vi "ConfigFilePath.vi"(11 "Model Name":string) -> (3 "appended path":path)   [LabVIEW 2025, in "DAQ_Module.lvlib" / "DAQ_Module.lvclass"]
uses:
  DAQ_Module.lvclass
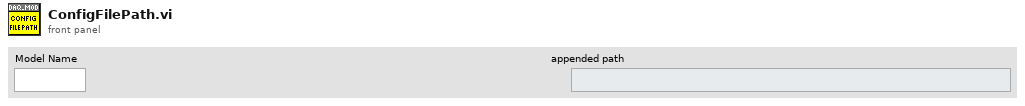
[diagram p1: front panel]
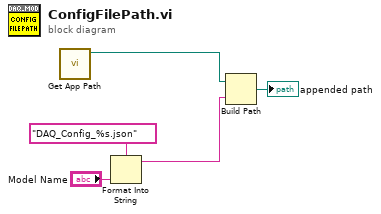
[diagram p0: block diagram]
diagram:
  n1 = call "Get App Path.vi"() -> ("Parent Directory (+ Relative)"=w4:path)  [unwired: 11 in]
  n2 = Format Into String(format string="DAQ_Config_%s.json", "Model Name") -> (resulting string=w2:string)  [unwired: 2 in, 1 out]
  n3 = Build Path(base path=w4, name or relative path=w2) -> (appended path=→"appended path":path)
